vi "4050_52_53_60_configure.vi"() -> ()   [LabVIEW 2010]
panel:
  in  "Port Name":string="MainNetwork"
  in  "Use checksum":bool
  in  "Baud Rate (9600)":u16(ring)=3 items=["1200 bps", "2400 bps", "4800 bps", "9600 bps", "19.2 kbps", "38.4 kbps"]
  out "Reply":string
  out "?":string
  in  "New Address":u8=200
  in  "Old Address":u8
  # "Leave off when in INIT*\nOtherwise use checksum"
  # "Happy reply starts \"!\"\nUnhappy reply starts \"?\""
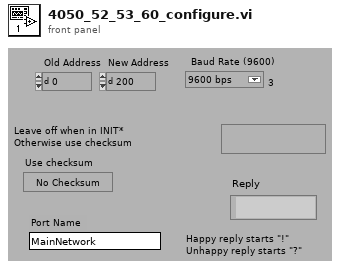
[diagram p1: front panel]
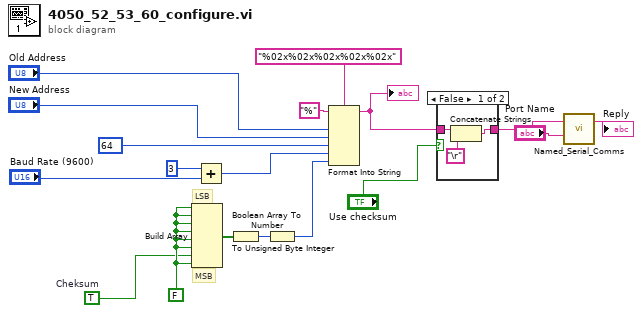
[diagram p0: block diagram]
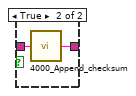
[diagram p2: hidden frame]
diagram:
  w1 = TRUE  # Cheksum
  w4 = FALSE
  # "MSB"
  # "LSB"
  n1 = Build Array(w4, w4, w4, w4, w4, w4, w1, w4) -> (w14:bool[])
  n2 = Add(x=u16 3, y="Baud Rate (9600)") -> (x+y=w8:u16)
  n3 = Boolean Array To Number(Boolean array=w14) -> (number=w13:u32)
  n4 = To Unsigned Byte Integer(number=w13) -> (unsigned 8bit integer=w12:u8)
  n5 = Format Into String(format string="%02x%02x%02x%02x%02x", initial string="%", "Old Address", "New Address", u16 64 ("Range Setting"), w8, w12) -> (resulting string=w11:string)  [unwired: 1 in, 1 out]
  "?" <- w11
  n6 = case shown="False" "Use checksum" {
    tunnel: w11 -> [w21 w23]
    tunnel: [w20 w22] -> w6
    frame False {
      n7 = Concatenate Strings(w21, "\r") -> (w20:string)
    }
    frame True {
      n8 = call "4000_Append_checksum.vi"("ADAM command"=w23) -> ("ADAM string to send"=w22:string)
    }
  }
  n9 = call "Named_Serial_Comms.vi"("Write String"=w6, "Port Name"="Port Name") -> ("Read"=→"Reply":string)  [unwired: 10 in, 3 out]
